vi "Get MetaData from Configurations.vi"(8 "error in":errorcluster, 11 "Configuration Cluster":variant) -> (0 "error out":errorcluster, 3 "configuration_parameters":T1[](array[typedef]))   [LabVIEW 2020, in "LineRegulation.lvlib"]
uses:
  LineRegulation.lvlib
  RPC Messages/ni_measurementlink_measurement_v1_ConfigurationParameter.ctl
  RPC Messages/ni_measurementlink_measurement_v1_ConfigurationParameter_AnnotationsEntry.ctl
  <vilib>/Utility/Data Type/NI_Data Type.lvlib
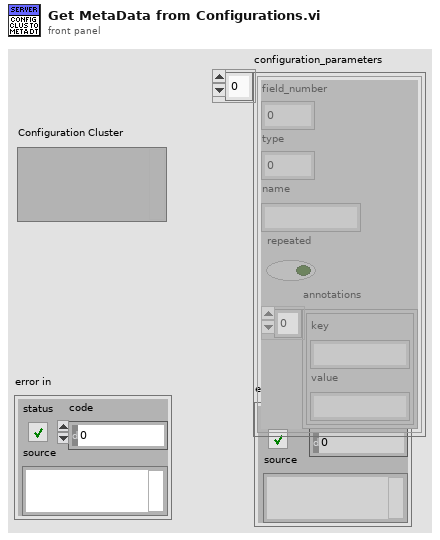
[diagram p1: front panel]
types:
  T1 = typedef "LineRegulation.lvlib/ni_measurementlink_measurement_v1_ConfigurationParameter.ctl" = cluster{"field_number":i32, "type":i32, "name":string, "repeated":bool, "annotations":T2[]}
  T2 = typedef "LineRegulation.lvlib/ni_measurementlink_measurement_v1_ConfigurationParameter_AnnotationsEntry.ctl" = cluster{"key":string, "value":string}
  T3 = cluster{"Parameter Name":string, "Annotations":cluster{"key":string, "value":string}[]}[]
  T4 = typedef "NI_Data Type.lvlib/Data Type.ctl" = enum8{"Invalid Type", "Void", "I8", "I16", "I32", "I64", "U8", "U16", "U32", "U64", "Single Float", "Double Float", "Extended Float", "Single Complex", "Double Complex", "Extended Complex", "Enum U8", "Enum U16", "Enum U32", "Enum U64", "Single Float With Unit", "Double Float With Unit", "Extended Float With Unit", "Single Complex with Unit", "Double Complex with Unit", "Extended Complex with Unit", "Boolean", "String", "Path", "Picture", "Tag", "Array", "Cluster", "Variant", "LV Variant", "Waveform", "Timestamp", "Digital Waveform", "Digital Data", "ExpressData", "Refnum", "External Data", "VI", "Poly VI", "LabVIEW Class Instance", "Fixed Point", "Set Collection", "Map Collection"}
  T5 = typedef "LineRegulation.lvlib/google_protobuf_Field_Kind.ctl" = enum32{"TYPE_UNKNOWN", "TYPE_DOUBLE", "TYPE_FLOAT", "TYPE_INT64", "TYPE_UINT64", "TYPE_INT32", "TYPE_FIXED64", "TYPE_FIXED32", "TYPE_BOOL", "TYPE_STRING", "TYPE_GROUP", "TYPE_MESSAGE", "TYPE_BYTES", "TYPE_UINT32", "TYPE_ENUM", "TYPE_SFIXED32", "TYPE_SFIXED64", "TYPE_SINT32", "TYPE_SINT64"}
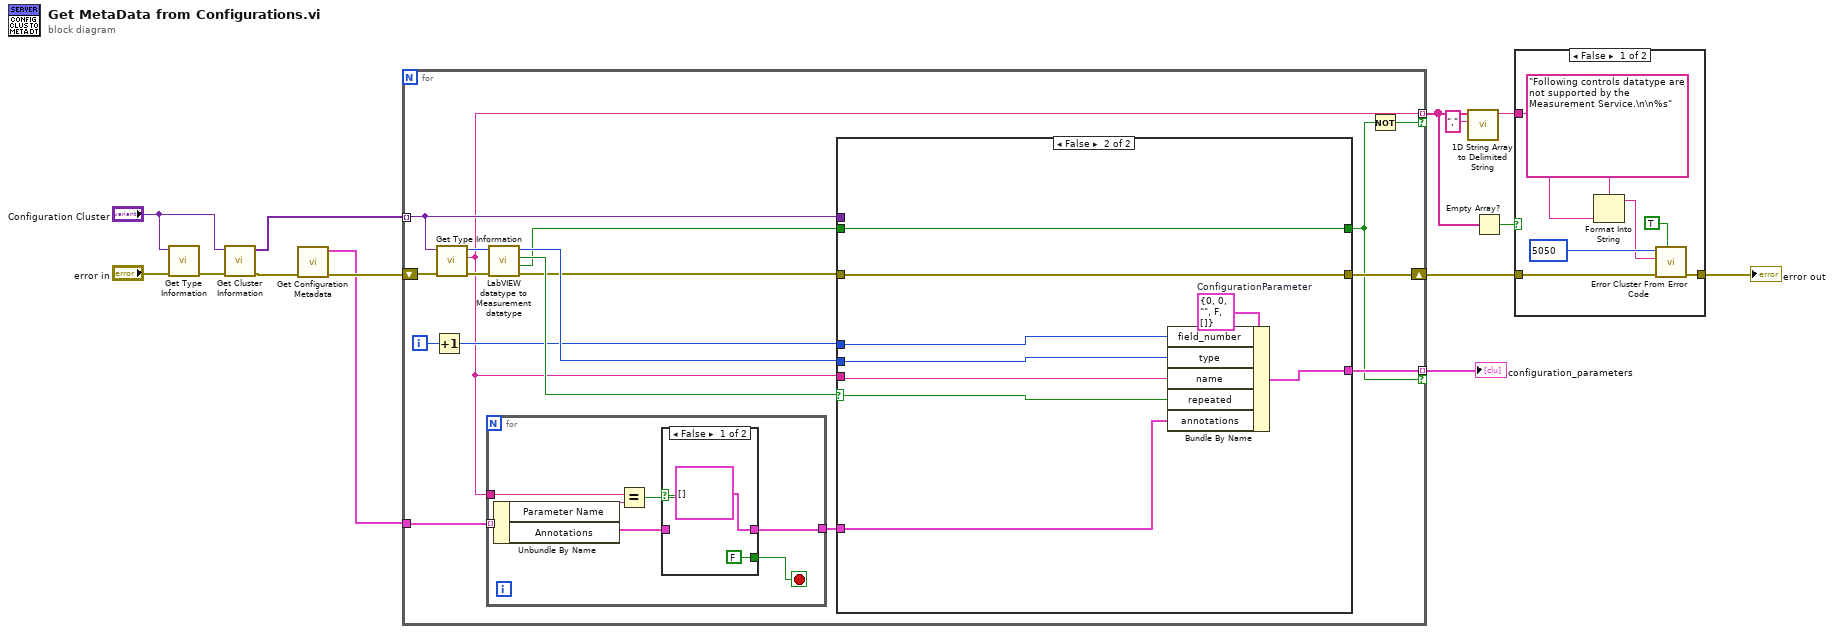
[diagram p0: block diagram]
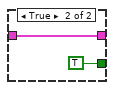
[diagram p3: hidden frame]
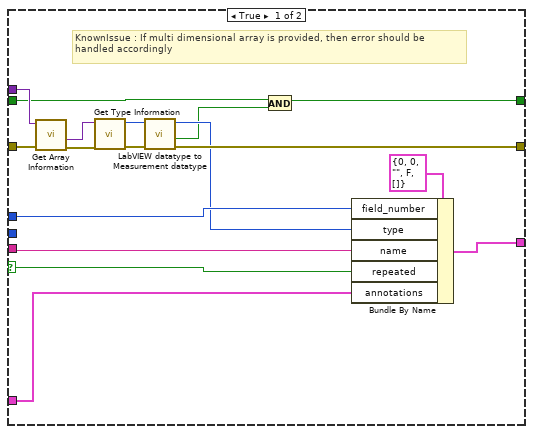
[diagram p4: hidden frame]
diagram:
  n1 = call <vilib>:"Get Type Information.vi"("error in (no error)"="error in", "variant"="Configuration Cluster") -> ("error out"=w14:errorcluster)  [unwired: 5 in, 4 out]
  n2 = call <vilib>:"Get Cluster Information.vi"("error in (no error)"=w14, "variant"="Configuration Cluster") -> ("error out"=w3:errorcluster, "cluster elements"=w13:variant[])  [unwired: 8 in]
  n3 = call "Get Configuration Metadata.vi"("error in (no error)"=w3) -> ("error out"=w2:errorcluster, "Metadata Value"=w1:T3)  [unwired: 9 in]
  n4 = for {
    tunnel: w13 -> [w25] mode=indexing
    tunnel: [w26] -> w12 mode=indexing if=w19
    shift-right: [w21] -> w10
    shift-left: w2 -> [w31]
    tunnel: [w16] -> w9 mode=indexing if=w18
    tunnel: w1 -> [w17]
    i -> [w30]
    n5 = Increment(x=w30) -> (x+1=w22:i32)
    n6 = call <vilib>:"Get Type Information.vi"("error in (no error)"=w31, "variant"=w25) -> ("error out"=w24:errorcluster, "name"=w16:string, "type"=w29:T4)  [unwired: 5 in, 2 out]
    n7 = for {
      tunnel: w17 -> [w37] mode=indexing
      tunnel: w16 -> [w38]
      tunnel: [w33] -> w15
      stop <- w32 stop-if-true
      n8 = Unbundle By Name(w37) -> ("Parameter Name"=w36:string, "Annotations"=w34:cluster{"key":string, "value":string}[])
      n9 = Equal?(x=w38, y=w36) -> (x = y?=w35:bool)
      n10 = case shown="False" w35 {
        tunnel: w34 -> [_ w42]
        tunnel: [cluster{"key":string, "value":string}[] [] ("Annotations") w42] -> w33
        tunnel: [FALSE TRUE] -> w32
        frame False {
        }
        frame True {
        }
      }
    }
    n11 = call "LabVIEW datatype to Measurement datatype.vi"("error in"=w24, "type"=w29) -> ("error out"=w23:errorcluster, "Supported?"=w20:bool, "Array?"=w27:bool, "MessageElementType"=w28:T5)  [unwired: 6 in]
    n12 = case shown="False" w27 {
      selector: w27 -> [w59 w68]
      tunnel: w22 -> [w49 w64]
      tunnel: w28 -> [_ w62]
      tunnel: [w58 w67] -> w26
      tunnel: w23 -> [w57 w66]
      tunnel: w25 -> [w56 _]
      tunnel: [w52 w66] -> w21
      tunnel: w16 -> [w47 w63]
      tunnel: w20 -> [w46 w61]
      tunnel: [w45 w61] -> w19
      tunnel: w15 -> [w43 w60]
      frame True {
        # "KnownIssue : If multi dimensional array is provided, then error should be handled accordingly"
        n13 = call <vilib>:"Get Array Information.vi"("error in (no error)"=w57, "variant"=w56) -> ("error out"=w55:errorcluster, "array element data type"=w51:variant)  [unwired: 6 in, 2 out]
        n14 = call <vilib>:"Get Type Information.vi"("error in (no error)"=w55, "variant"=w51) -> ("error out"=w53:errorcluster, "type"=w54:T4)  [unwired: 5 in, 3 out]
        n15 = call "LabVIEW datatype to Measurement datatype.vi"("error in"=w53, "type"=w54) -> ("error out"=w52:errorcluster, "Supported?"=w44:bool, "MessageElementType"=w48:T5)  [unwired: 6 in, 1 out]
        n16 = And(x=w46, y=w44) -> (x .and. y?=w45:bool)
        n17 = Bundle By Name(cluster=T1 {"field_number"=0, "type"=0, "name"="", "repeated"=FALSE, "annotations"=[]} ("ConfigurationParameter"), "field_number"=w49, "type"=w48, "name"=w47, "repeated"=w59, "annotations"=w43) -> (w58:T1)
      }
      frame False {
        w65 = T1 {"field_number"=0, "type"=0, "name"="", "repeated"=FALSE, "annotations"=[]}  # ConfigurationParameter
        n18 = Bundle By Name(cluster=w65, "field_number"=w64, "type"=w62, "name"=w63, "repeated"=w68, "annotations"=w60) -> (w67:T1)
      }
    }
    n19 = Not(x=w19) -> (.not. x?=w18:bool)
  }
  "configuration_parameters" <- w12
  n20 = call <vilib>:"1D String Array to Delimited String.vi"("delimiter"=",", "string array"=w9) -> ("delimited string"=w7:string)  [unwired: 9 in]
  n21 = Empty Array?(array=w9) -> (empty?=w8:bool)
  n22 = case shown="False" w8 {
    tunnel: w10 -> [w75 w76]
    tunnel: [w74 w76] -> w4
    tunnel: w7 -> [w71 _]
    frame False {
      n23 = Format Into String(format string="Following controls datatype are not supported by the Measurement Service.\n\n%s", w71) -> (resulting string=w70:string)  [unwired: 2 in, 1 out]
      n24 = call <vilib>:"Error Cluster From Error Code.vi"("show call chain? (False)"=TRUE, "error in (no error)"=w75, "error message (\"\")"=w70, "error code (0)"=5050) -> ("error out"=w74:errorcluster)  [unwired: 5 in]
    }
    frame True {
    }
  }
  "error out" <- w4
